vi "Array to Cluster.vi"(8 "Error In":errorcluster, 9 "Input String":string, 10 "array":dbl[](array[numeric])) -> (0 "Error Out":errorcluster, 1 "Output":cluster{"Y":dbl[]}[](array[cluster]), 2 "Output Label":string[](array[string]))   [LabVIEW 2016]
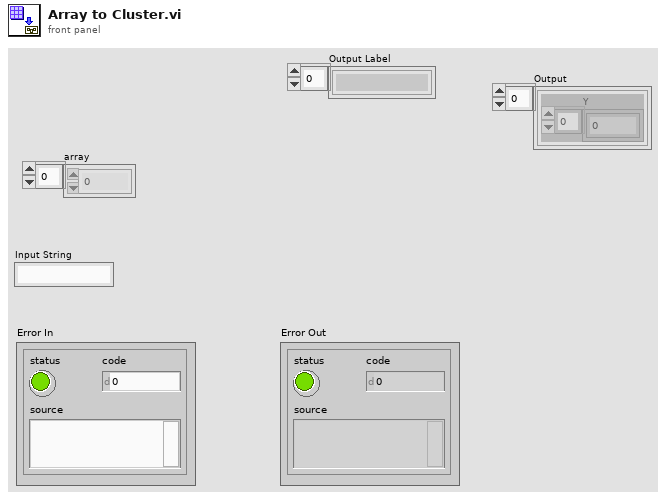
[diagram p1: front panel]
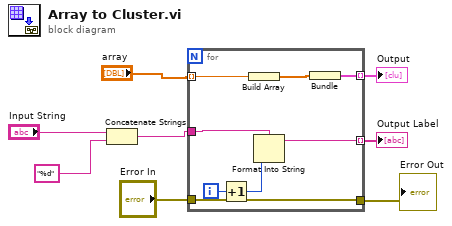
[diagram p0: block diagram]
diagram:
  n1 = Concatenate Strings("Input String", "%d" ("wavenames")) -> (w6:string)
  n2 = for {
    tunnel: [w15] -> w4 mode=indexing
    tunnel: [w13] -> w5 mode=indexing
    tunnel: w6 -> [w12]
    tunnel: "array" -> [w10] mode=indexing
    tunnel: "Error In" -> [w11]
    tunnel: [w11] -> w2
    i -> [w16]
    n3 = Increment(x=w16) -> (x+1=w14:i32)
    n4 = Build Array(w10) -> (w9:dbl[])
    n5 = Format Into String(format string=w12, w14) -> (resulting string=w15:string)  [unwired: 2 in, 1 out]
    n6 = Bundle(w9) -> (w13:cluster{dbl[]})  [unwired: 1 in]
  }
  "Output" <- w5
  "Output Label" <- w4
  "Error Out" <- w2
